vi "HW Starus.vi"(8 "error in":errorcluster, 9 "Status":bool, 10 "HW Module":T1) -> (0 "error out":errorcluster)   [LabVIEW 2024, in "Controller.lvlib"]
doc: "_____\nCreated using DQMH Framework: Event Scripter 7.1.0.1503.\n\n_____\nCreated using DQMH Framework: Event Scripter 7.1.0.1503."
uses:
  Controller.lvlib
  GUI/Controls/HW Modules.ctl
  HW Starus Argument--cluster.ctl
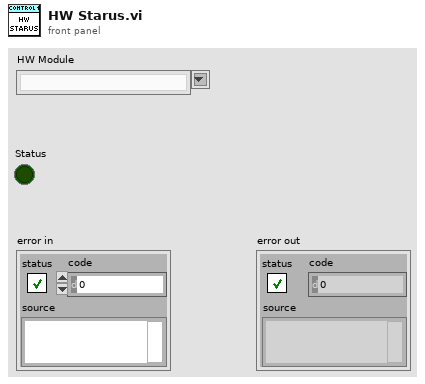
[diagram p1: front panel]
types:
  T1 = typedef "HW Modules.ctl" = string
  T2 = typedef "Controller.lvlib/HW Starus Argument--cluster.ctl" = cluster{"HW Module":T1, "Status":bool}
  T3 = typedef "Controller.lvlib/Request Events--cluster.ctl" = cluster{"Stop Module":refnum<user-event>, "Show Panel":refnum<user-event>, "Hide Panel":refnum<user-event>, "Get Module Execution Status":refnum<user-event>, "Show Diagram":refnum<user-event>, "Login":refnum<user-event>, "Logout":refnum<user-event>, "scanner data received":refnum<user-event>, "connect all modules":refnum<user-event>, "HW Starus":refnum<user-event>}
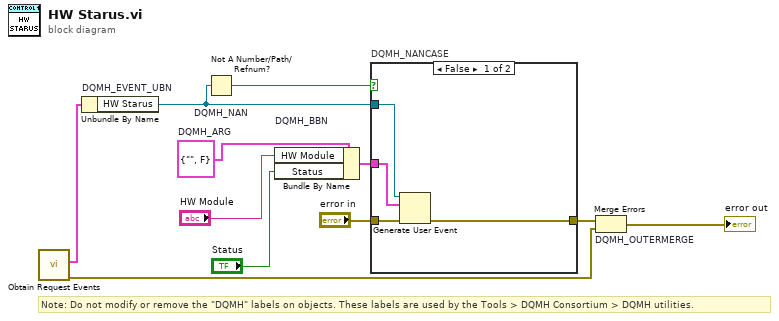
[diagram p0: block diagram]
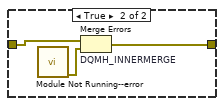
[diagram p2: hidden frame]
diagram:
  w5 = T2 {"HW Module"="", "Status"=FALSE}  # DQMH_ARG
  # "Note: Do not modify or remove the \"DQMH\" labels on objects. These labels are used by the Tools > DQMH Consortium > DQMH utilities."
  n1 = call "Obtain Request Events.vi"() -> ("error out"=w2:errorcluster, "Controller Request Events"=w1:T3)  [unwired: 10 in]
  n2 = Unbundle By Name "DQMH_EVENT_UBN"(w1) -> ("HW Starus"=w7:refnum<user-event>)
  n3 = Not A Number/Path/Refnum? "DQMH_NAN"(number/path/refnum=w7) -> (NaN/Path/Refnum?=w8:bool)
  n4 = Bundle By Name "DQMH_BBN"(cluster=w5, "HW Module"="HW Module", "Status"="Status") -> (w9:T2)
  n5 = case "DQMH_NANCASE" shown="False" w8 {
    tunnel: "error in" -> [w15 w18]
    tunnel: [w14 w17] -> w6
    tunnel: w7 -> [w13 _]
    tunnel: w9 -> [w12 _]
    frame False {
      n6 = Generate User Event(user event=w13, event data cluster=w12, error in=w15) -> (error out=w14:errorcluster)  [unwired: 1 in, 1 out]
    }
    frame True {
      n7 = call "Module Not Running--error.vi"() -> ("error out"=w16:errorcluster)  [unwired: 11 in]
      n8 = Merge Errors "DQMH_INNERMERGE"(w18, w16) -> (w17:errorcluster)
    }
  }
  n9 = Merge Errors "DQMH_OUTERMERGE"(w6, w2) -> (→"error out":errorcluster)
